vi "Initialize Data.vi"(8 "error in (no error)":errorcluster, 9 "data version":T1, 10 "data":string, 11 "Core Groups Configuration in":refnum<class "Core Groups Configuration.lvclass">) -> (0 "error out":errorcluster, 3 "Core Groups Configuration out":refnum<class "Core Groups Configuration.lvclass">)   [LabVIEW 2017, in "DSF Core.lvlib" / "Core Groups Configuration.lvclass"]
uses:
  Core Groups Configuration.lvclass
  Typedefs/DSF Version Info.ctl
  Core Groups Configuration.lvclass/Core Groups Configuration.ctl
  DSF Core.lvlib
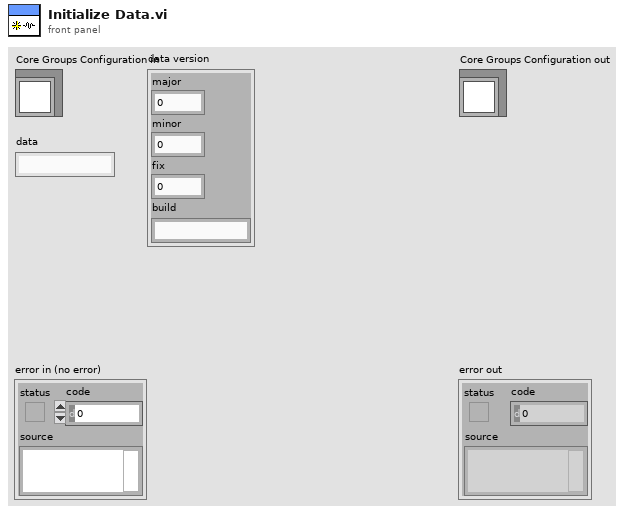
[diagram p1: front panel]
types:
  T1 = typedef "DSF Core.lvlib/DSF Version Info.ctl" = cluster{"major":i32, "minor":i32, "fix":i32, "build":string}
  T2 = cluster{"name":string, "direction":u8, "cycle timing":cluster{"priority":u64, "decimation":u64, "offset":u64}, "timeout behavior":u8, "convert buffers":bool}[]
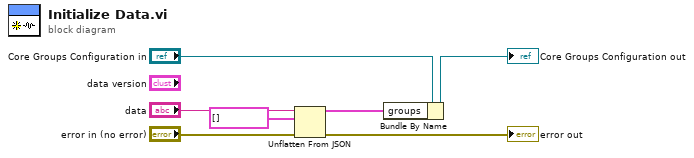
[diagram p0: block diagram]
diagram:
  n1 = Unflatten From JSON(JSON string="data", type and defaults=T2 [] ("Cluster"), error in (no error)="error in (no error)") -> (value=w4:T2, error out=→"error out":errorcluster)  [unwired: 4 in]
  n2 = Bundle By Name(cluster="Core Groups Configuration in", "groups"=w4) -> (→"Core Groups Configuration out":refnum<class "Core Groups Configuration.lvclass">)
